vi "testTemp.vi"() -> ()   [LabVIEW 2017]
uses:
  <vilib>/Utility/file.llb/Write Delimited Spreadsheet (I64).vi
panel:
  in  "Rat 2":string
  in  "Rat":string
  in  "choices":i32[][](array[numeric])
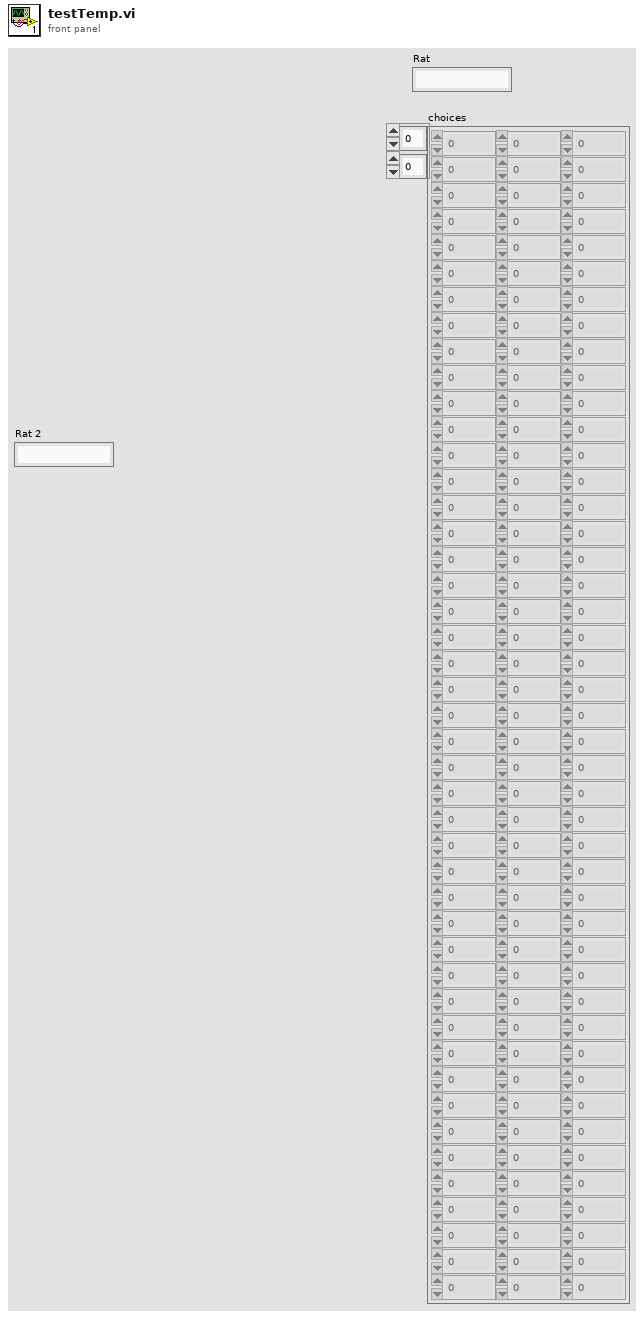
[diagram p1: front panel]
types:
  T1 = enum16{"big-endian, network order", "native, host order", "little-endian"}
  T2 = enum16{"open", "replace", "create", "open or create", "replace or create", "replace or create with confirmation"}
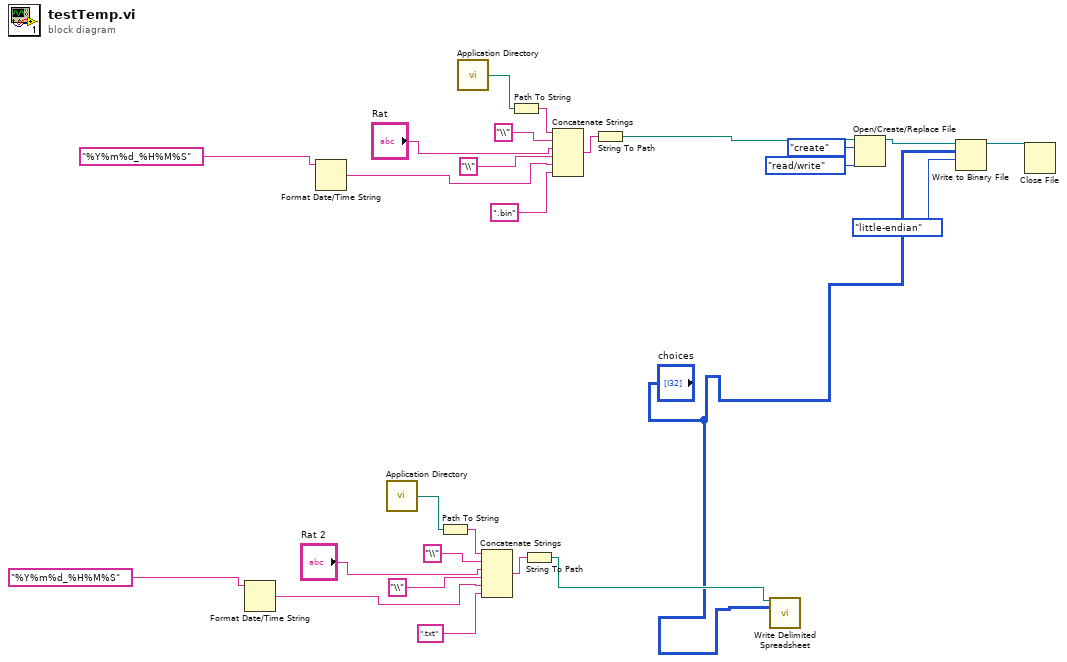
[diagram p0: block diagram]
diagram:
  n1 = Format Date/Time String(time format string (%c)="%Y%m%d_%H%M%S" ("time string")) -> (date/time string=w5:string)  [unwired: 2 in]
  n2 = Format Date/Time String(time format string (%c)="%Y%m%d_%H%M%S" ("time string")) -> (date/time string=w20:string)  [unwired: 2 in]
  n3 = call <vilib>:"Application Directory.vi"() -> ("Application Directory"=w3:path)
  n4 = Path To String(path=w3) -> (string=w11:string)
  n5 = call <vilib>:"Application Directory.vi"() -> ("Application Directory"=w18:path)
  n6 = Concatenate Strings(w11, "\\" ("string"), "Rat 2", "\\" ("string"), w5, ".txt") -> (w10:string)
  n7 = Path To String(path=w18) -> (string=w26:string)
  n8 = String To Path(string=w10) -> (path=w2:path)
  n9 = Concatenate Strings(w26, "\\" ("string"), "Rat", "\\" ("string"), w20, ".bin") -> (w25:string)
  n10 = String To Path(string=w25) -> (path=w13:path)
  n11 = call-poly <vilib>:"Write Delimited Spreadsheet.vi"("file path (dialog if empty)"=w2, "2D data"="choices") -> ()  [unwired: 12 in, 2 out]
  n12 = Open/Create/Replace File(file path (use dialog)=w13, operation (0:open)=T2."create", access (0:read/write)=enum16{"read/write", "read-only", "write-only"}."read/write") -> (refnum out=w15:refnum<file>)  [unwired: 3 in, 2 out]
  n13 = Write to Binary File(file (use dialog)=w15, data="choices", 9:T1."little-endian" ("byte order (0:big-endian, network order)")) -> (refnum out=w12:refnum<file>)  [unwired: 3 in, 2 out]
  n14 = Close File(refnum=w12) -> ()  [unwired: 1 in, 2 out]
